vi "serenial.io-ase fix shared library paths.vi"(8 "error in":errorcluster, 10 "class path":path, 11 "Shared Library Path":path caption="Shared Library Path - bitness and extn will be replaced with wildcards") -> (0 "error out":errorcluster)   [LabVIEW 2024]
uses:
  <vilib>/Utility/traverseref.llb/TRef TravTarget.ctl
  <vilib>/Utility/traverseref.llb/VI Scripting - Traverse.lvlib
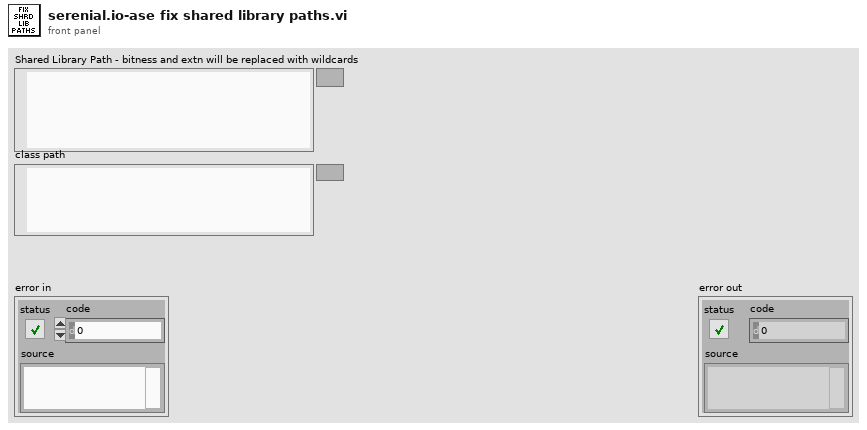
[diagram p1: front panel]
types:
  T1 = typedef "TRef TravTarget.ctl" = enum16{"FP", "BD", "Other"}
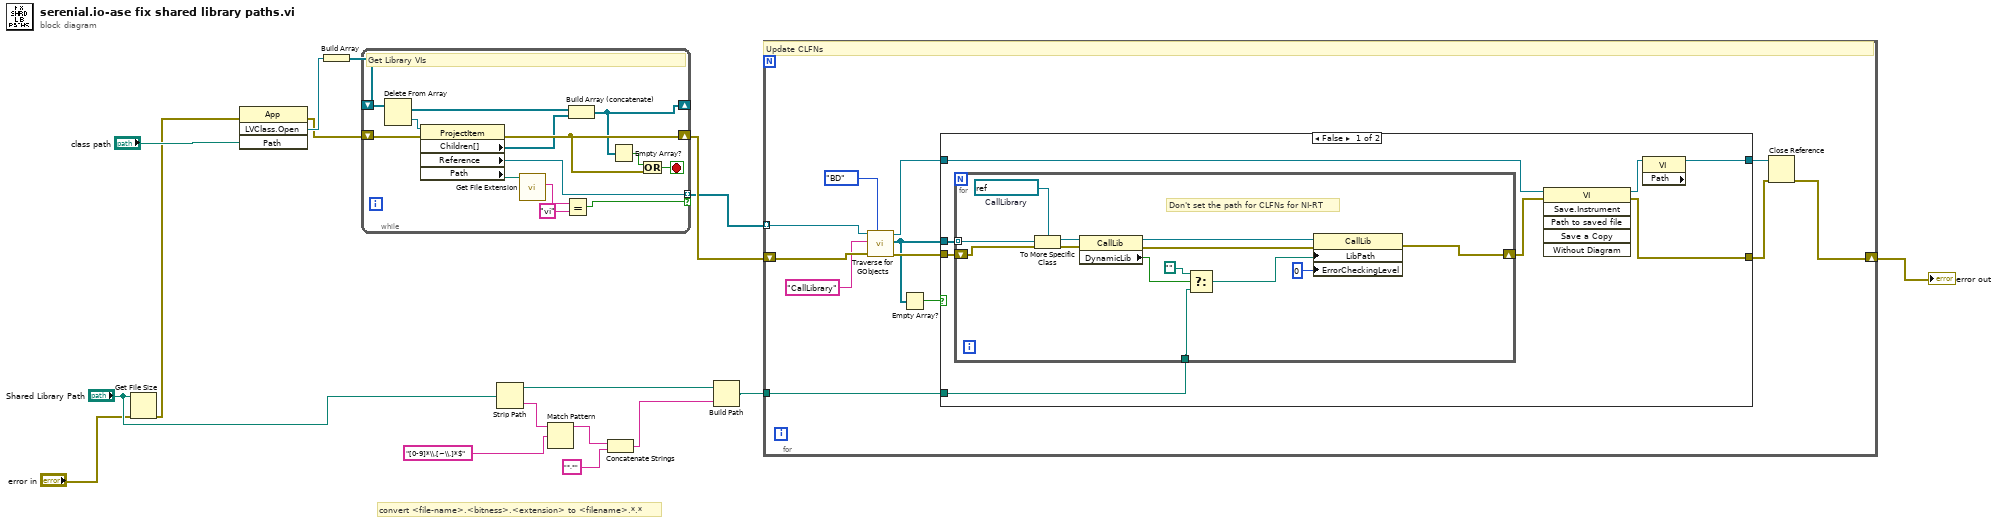
[diagram p0: block diagram]
diagram:
  # "convert <file-name>.<bitness>.<extension> to <filename>.*.*"
  n1 = Get File Size(file="Shared Library Path", error in="error in") -> (0:w1:errorcluster)  [unwired: 2 out]
  n2 = invoke class="App" method="LVClass.Open"(error in=w1, "Path"="class path") -> (error out=w15:errorcluster, "LVClass.Open"=w16:refnum<vi>)  [unwired: 2 in, 2 out]
  n3 = Build Array(w16) -> (w14:refnum<vi>[])
  n4 = while {
    shift-right: [w26] -> w13
    shift-left: w15 -> [w31]
    shift-right: [w22] -> _
    shift-left: w14 -> [w30]
    tunnel: [w23] -> w12 mode=indexing if=w18
    stop <- w27 stop-if-true
    # "Get Library VIs"
    n5 = Delete From Array(array=w30) -> (deleted portion=w25:refnum<vi>, array with subset deleted=w29:refnum<vi>[])  [unwired: 2 in]
    n6 = property class="ProjectItem"(reference=w25, error in=w31) -> (error out=w26:errorcluster, "Children[]"=w24:refnum<vi>[], "Reference"=w23:refnum<vi>, "Path"=w19:path)  [unwired: 1 out]
    n7 = call <vilib>:"Get File Extension.vi"("file"=w19) -> ("lowercase file extension"=w21:string)  [unwired: 6 in, 4 out]
    n8 = Equal?(x=w21, y="vi") -> (x = y?=w18:bool)
    n9 = Build Array (concatenate)(w29, w24) -> (w22:refnum<vi>[])
    n10 = Empty Array?(array=w22) -> (empty?=w28:bool)
    n11 = Or(x=w28, y=w26) -> (x .or. y?=w27:bool)
  }
  n12 = Strip Path(path="Shared Library Path") -> (stripped path=w3:path, name=w8:string)
  n13 = Match Pattern(string=w8, regular expression="[0-9]*\\.[~\\.]*$") -> (before substring=w6:string)  [unwired: 1 in, 3 out]
  n14 = Concatenate Strings(w6, "*.*" ("format string")) -> (w4:string)
  n15 = Build Path(base path=w3, name or relative path=w4) -> (appended path=w11:path)
  n16 = for {
    shift-right: [w43] -> w17
    shift-left: w13 -> [w41]
    tunnel: w11 -> [w42]
    tunnel: w12 -> [w40] mode=indexing
    # "Update CLFNs"
    n17 = call <vilib>:"Traverse for GObjects.vi"("Traverse Target"=TRef_TravTarget."BD", "error in (no error)"=w41, "Class Name"="CallLibrary", "VI Refnum"=w40) -> ("error out"=w37:errorcluster, "References"=w35:refnum<vi>[], "dup VI Refnum"=w36:refnum<vi>)  [unwired: 4 in, 1 out]
    n18 = Empty Array?(array=w35) -> (empty?=w32:bool)
    n19 = case shown="False" w32 {
      tunnel: w37 -> [w51 w65]
      tunnel: w36 -> [w50 w66]
      tunnel: w35 -> [w49 _]
      tunnel: [w44 w66] -> w34
      tunnel: [w46 w65] -> w33
      tunnel: w42 -> [w45 _]
      frame False {
        n20 = for {
          tunnel: w49 -> [w64] mode=indexing
          shift-right: [w60] -> w48
          shift-left: w51 -> [w62]
          tunnel: w45 -> [w52]
          w63 = refnum<vi> refnum  # CallLibrary
          # "Don't set the path for CLFNs for NI-RT"
          n21 = To More Specific Class(target class=w63, reference=w64, error in=w62) -> (specific class reference=w61:refnum<vi>, error out=w58:errorcluster)
          n22 = property class="CallLib"(reference=w61, error in=w58) -> (reference out=w59:refnum<vi>, error out=w57:errorcluster, "DynamicLib"=w56:bool)
          n23 = Select(t=path "", s=w56, f=w52) -> (s? t:f=w53:path)
          n24 = property class="CallLib"(reference=w59, error in=w57, "LibPath"=w53, "ErrorCheckingLevel"=u32 0 ("Error Checking Level")) -> (error out=w60:errorcluster)  [unwired: 1 out]
        }
        n25 = invoke class="VI" method="Save.Instrument"(reference=w50, error in=w48) -> (reference out=w47:refnum<vi>, error out=w46:errorcluster)  [unwired: 4 in, 4 out]
        n26 = property class="VI" props=["Path"](reference=w47) -> (reference out=w44:refnum<vi>)  [unwired: 1 in, 2 out]
      }
      frame True {
      }
    }
    n27 = Close Reference(reference=w34, error in (no error)=w33) -> (error out=w43:errorcluster)
  }
  "error out" <- w17
